vi "CompassRefNum_Simulation_Global.vi"(0 "menu":enum16{"set", "get", "delete"}(ring)=enum."get", 7 "Analog Channel":T1=enum."AI 1", 9 "Honeywell Compass HMC6343 Set":refnum<class "Honeywell Compass HMC6343.lvclass">, 11 "error in (no error)":errorcluster) -> (10 "Honeywell Compass HMC6343 Get":refnum<class "Honeywell Compass HMC6343.lvclass">, 15 "error out":errorcluster)   [LabVIEW 2017]
doc: "Sets a reference into a registry, gets a reference from a registry, or deletes a reference from a registry. The reference is accessed by name, and can be given any unique name.\n\nThis software is licensed. Open the labview\\readme\\WPI Robotics Library Open Source License.txt file for more information."
uses:
  <vilib>/Rock Robotics/SystemInterfaces/AI/FPGA_AIGyroChannel.ctl
  <instrlib>/Honeywell Compass HMC6343/HAIOL/Honeywell Compass HMC6343.lvclass
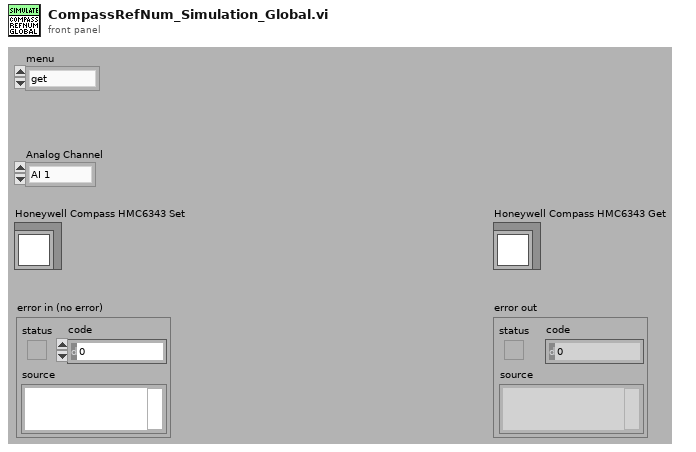
[diagram p1: front panel]
types:
  T1 = typedef "FPGA_AIGyroChannel.ctl" = enum8{"AI 0", "AI 1", "Invalid"}
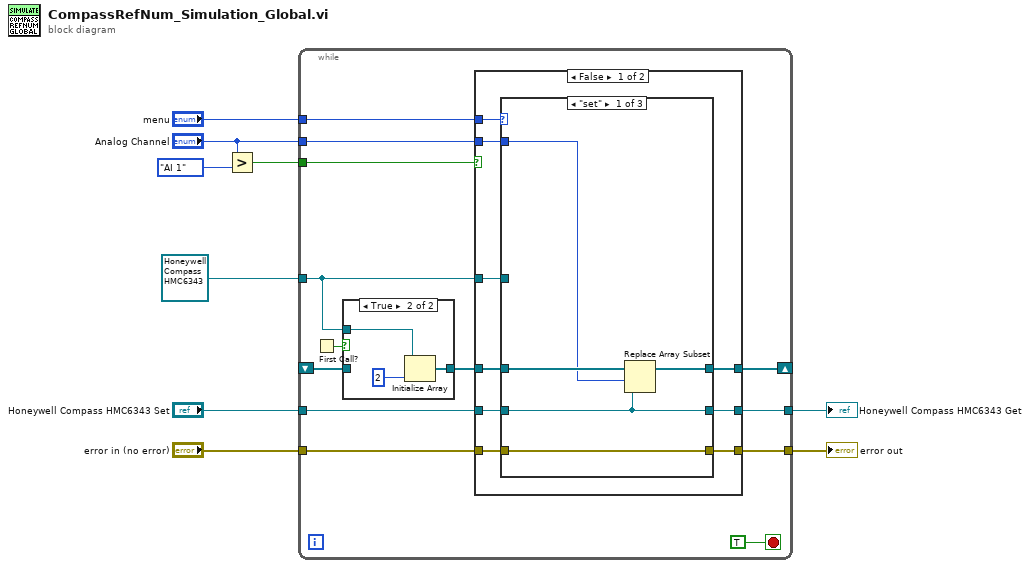
[diagram p0: block diagram]
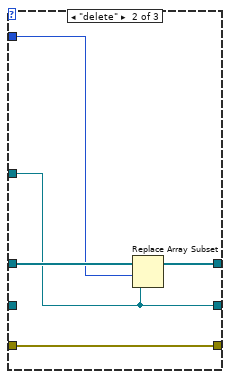
[diagram p2: hidden frame]
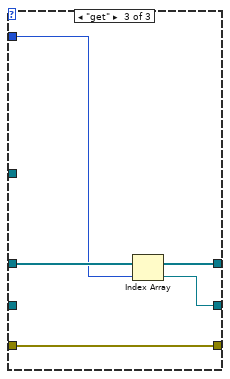
[diagram p3: hidden frame]
diagram:
  n1 = Greater?(x="Analog Channel", y=FPGA_AIGyroChannel."AI 1") -> (0:w1:bool)
  n2 = while {
    tunnel: "Honeywell Compass HMC6343 Set" -> [w22]
    tunnel: "error in (no error)" -> [w18]
    shift-right: [w21] -> _
    shift-left: _ -> [w13]
    tunnel: [w20] -> w3
    tunnel: "menu" -> [w19]
    tunnel: [w17] -> w8
    tunnel: "Analog Channel" -> [w12]
    tunnel: w1 -> [w11]
    tunnel: refnum<class "Honeywell Compass HMC6343.lvclass"> refnum ("Honeywell Compass HMC6343 Get") -> [w10]
    stop <- TRUE stop-if-true
    n3 = First Call?() -> (First Call?: T/F=w15:bool)
    n4 = case shown="True" w15 {
      tunnel: [w49 w51] -> w14
      tunnel: w13 -> [w49 _]
      tunnel: w10 -> [_ w50]
      frame False {
      }
      frame True {
        n5 = Initialize Array(w50, 2 ("dimension size")) -> (w51:refnum<class "Honeywell Compass HMC6343.lvclass">[])
      }
    }
    n6 = case shown="False" w11 {
      tunnel: w22 -> [w31 _]
      tunnel: [w30 w48] -> w21
      tunnel: [w29 w46] -> w20
      tunnel: w19 -> [w28 _]
      tunnel: w18 -> [w27 w47]
      tunnel: [w26 w47] -> w17
      tunnel: w14 -> [w25 w48]
      tunnel: w12 -> [w24 _]
      tunnel: w10 -> [w23 w46]
      frame False {
        n7 = case shown="\"set\"" w28 {
          tunnel: w31 -> [w34 _ _]
          tunnel: [w35 w40 w45] -> w30
          tunnel: w25 -> [w36 w41 w45]
          tunnel: [w34 w37 w44] -> w29
          tunnel: [w33 w39 w43] -> w26
          tunnel: w27 -> [w33 w39 w43]
          tunnel: w24 -> [w32 w38 w42]
          tunnel: w23 -> [_ w37 _]
          frame "set" {
            n8 = Replace Array Subset(array=w36, new element=w34, index=w32) -> (w35:refnum<class "Honeywell Compass HMC6343.lvclass">[])
          }
          frame "delete" {
            n9 = Replace Array Subset(array=w41, new element=w37, index=w38) -> (w40:refnum<class "Honeywell Compass HMC6343.lvclass">[])
          }
          frame "get" {
            n10 = Index Array(array=w45, index=w42) -> (element=w44:refnum<class "Honeywell Compass HMC6343.lvclass">)
          }
        }
      }
      frame True {
        # "Do nothing if channel is Invalid."
      }
    }
  }
  "error out" <- w8
  "Honeywell Compass HMC6343 Get" <- w3
